vi "FTW-Crypto-PublicKeySignature-Verify.vi"(0 "Data":string="Data to encrypt!", 5 "Hex Encoded Signature":string, 7 "Public Key":string, 11 "error in":errorcluster) -> (4 "Signature Verified":bool, 15 "error out":errorcluster)   [LabVIEW 2015]
panel:
  # "Inputs"
  # "Outputs"
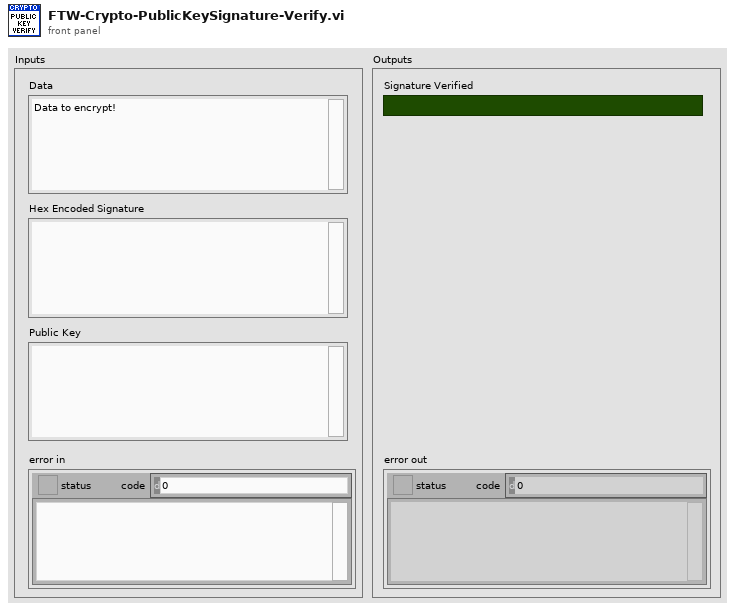
[diagram p1: front panel]
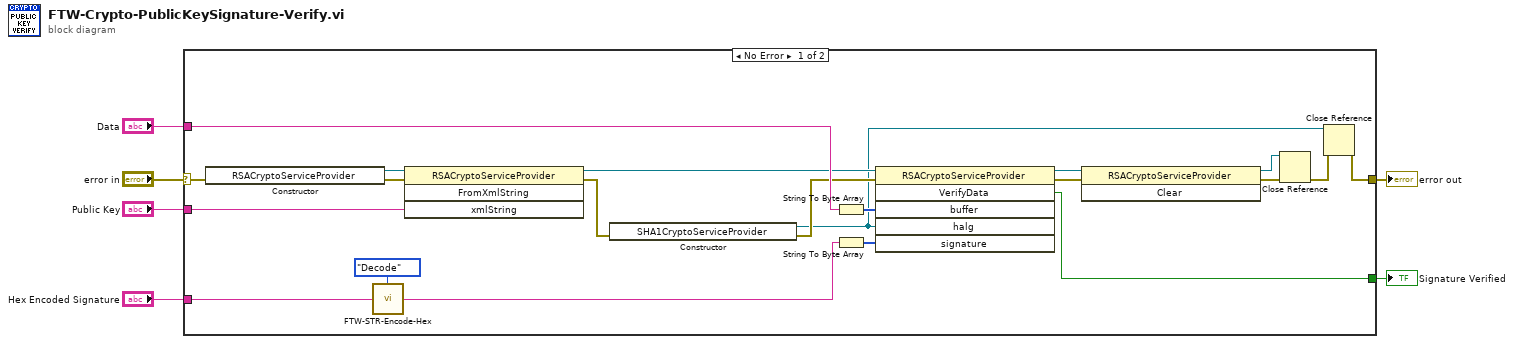
[diagram p0: block diagram]
diagram:
  n1 = case shown="No Error" "error in" {
    selector: "error in" -> [w27 w28]
    tunnel: "Data" -> [w26 _]
    tunnel: "Hex Encoded Signature" -> [w15 _]
    tunnel: [w7 w28] -> w3
    tunnel: [w23 _] -> w2
    tunnel: "Public Key" -> [w17 _]
    frame No Error {
      n2 = constructor class="RSACryptoServiceProvider"(error in=w27) -> (reference out=w21:refnum<k24>, error out=w19:errorcluster)  [unwired: 2 in, 1 out]
      n3 = call "FTW-STR-Encode-Hex.vi"("Input"=w15, "Direction"=enum16{"Encode", "Decode"}."Decode") -> ("Output"=w14:string)
      n4 = invoke class="RSACryptoServiceProvider" method="FromXmlString"(reference=w21, error in=w19, "xmlString"=w17) -> (reference out=w20:refnum<k24>, error out=w18:errorcluster)  [unwired: 1 in, 2 out]
      n5 = constructor class="SHA1CryptoServiceProvider"(error in=w18) -> (reference out=w9:refnum<k24>, error out=w24:errorcluster)  [unwired: 2 in, 1 out]
      n6 = String To Byte Array(string=w26) -> (unsigned byte array=w25:u8[])
      n7 = String To Byte Array(string=w14) -> (unsigned byte array=w22:u8[])
      n8 = invoke class="RSACryptoServiceProvider" method="VerifyData"(reference=w20, error in=w24, "buffer"=w25, "halg"=w9, "signature"=w22) -> (reference out=w13:refnum<k24>, error out=w12:errorcluster, "VerifyData"=w23:bool)  [unwired: 1 in, 3 out]
      n9 = invoke class="RSACryptoServiceProvider" method="Clear"(reference=w13, error in=w12) -> (reference out=w11:refnum<k24>, error out=w10:errorcluster)  [unwired: 1 in, 1 out]
      n10 = Close Reference(reference=w11, error in (no error)=w10) -> (error out=w8:errorcluster)
      n11 = Close Reference(reference=w9, error in (no error)=w8) -> (error out=w7:errorcluster)
    }
    frame Error {
    }
  }
  "error out" <- w3
  "Signature Verified" <- w2
